vi "Move Main VI Controls.vi"(8 "error in":errorcluster, 11 "VIRef in":refnum<vi>) -> (0 "error out":errorcluster)   [LabVIEW 2018]
uses:
  <vilib>/Utility/miscctls.llb/LVPointTypeDef.ctl
panel:
  out "Height":i16
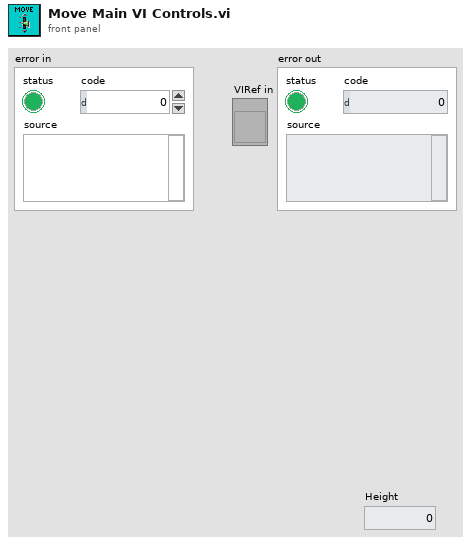
[diagram p1: front panel]
types:
  T1 = typedef "LVPointTypeDef.ctl" = cluster{"Horizontal":i16, "Vertical":i16}
  T2 = typedef "LVRectTypeDef.ctl" = cluster{"Left":i16, "Top":i16, "Right":i16, "Bottom":i16}
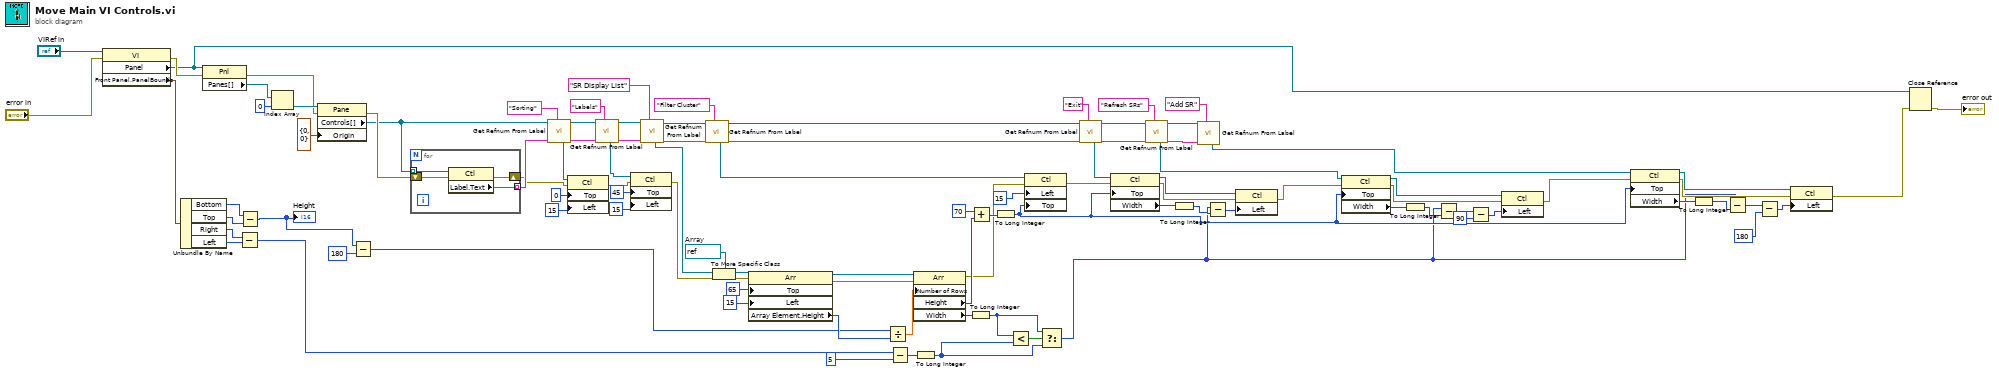
[diagram p0: block diagram]
diagram:
  w69 = refnum<vi> refnum  # Array
  n1 = property class="VI"(reference="VIRef in", error in="error in") -> (error out=w95:errorcluster, "Panel"=w9:refnum<vi>, "Front Panel.PanelBounds"=w92:T2)  [unwired: 1 out]
  n2 = Unbundle By Name(w92) -> ("Bottom"=w57:i16, "Top"=w56:i16, "Right"=w47:i16, "Left"=w46:i16)
  n3 = property class="Pnl"(reference=w9, error in=w95) -> (error out=w94:errorcluster, "Panes[]"=w96:refnum<vi>[])  [unwired: 1 out]
  n4 = Subtract(x=w47, y=w46) -> (x-y=w19:i16)
  n5 = Subtract(x=w57, y=w56) -> (x-y=w54:i16)
  "Height" <- w54
  n6 = Index Array(array=w96, index=0) -> (element=w97:refnum<vi>)
  n7 = property class="Pane"(reference=w97, error in=w94, "Origin"=T1 {"Horizontal"=0, "Vertical"=0}) -> (error out=w93:errorcluster, "Controls[]"=w90:refnum<vi>[])  [unwired: 1 out]
  n8 = Subtract(x=w54, y=i16 180) -> (x-y=w53:i16)
  n9 = for {
    tunnel: w90 -> [w102] mode=indexing
    shift-right: [w103] -> w62
    shift-left: w93 -> [w104]
    tunnel: [w101] -> w89 mode=indexing
    n10 = property class="Ctl"(reference=w102, error in=w104) -> (error out=w103:errorcluster, "Label.Text"=w101:string)  [unwired: 1 out]
  }
  n11 = call "Get Refnum From Label.vi"("label"="Sorting" ("element"), "label array in"=w89, "controls[] in"=w90) -> ("label array out"=w86:string[], "controls[] out"=w87:refnum<vi>[], "refnum out"=w72:refnum<vi>)  [unwired: 6 in]
  n12 = property class="Ctl"(reference=w72, error in=w62, "Top"=0 ("Position:Left"), "Left"=15 ("Position:Top")) -> (error out=w65:errorcluster)  [unwired: 1 out]
  n13 = call "Get Refnum From Label.vi"("label"="Labels" ("element"), "label array in"=w86, "controls[] in"=w87) -> ("label array out"=w83:string[], "controls[] out"=w84:refnum<vi>[], "refnum out"=w71:refnum<vi>)  [unwired: 6 in]
  n14 = property class="Ctl"(reference=w71, error in=w65, "Top"=45 ("Position:Top"), "Left"=15 ("Position:Left")) -> (error out=w64:errorcluster)  [unwired: 1 out]
  n15 = call "Get Refnum From Label.vi"("label"="SR Display List" ("element"), "label array in"=w83, "controls[] in"=w84) -> ("label array out"=w85:string[], "controls[] out"=w82:refnum<vi>[], "refnum out"=w3:refnum<vi>)  [unwired: 6 in]
  n16 = call "Get Refnum From Label.vi"("label"="Filter Cluster" ("element"), "label array in"=w85, "controls[] in"=w82) -> ("label array out"=w5:string[], "controls[] out"=w4:refnum<vi>[], "refnum out"=w52:refnum<vi>)  [unwired: 6 in]
  n17 = To More Specific Class(target class=w69, reference=w3, error in=w64) -> (specific class reference=w2:refnum<vi>, error out=w63:errorcluster)
  n18 = property class="Arr"(reference=w2, error in=w63, "Top"=65 ("Position:Top"), "Left"=15 ("Position:Left")) -> (reference out=w60:refnum<vi>, error out=w6:errorcluster, "Array Element.Height"=w59:u32)
  n19 = Divide(x=w53, y=w59) -> (x/y=w58:dbl)
  n20 = Subtract(x=w19, y=i16 5) -> (x-y=w16:i16)
  n21 = property class="Arr"(reference=w60, error in=w6, "Number of Rows"=w58) -> (error out=w45:errorcluster, "Height"=w50:u32, "Width"=w17:u32)  [unwired: 1 out]
  n22 = To Long Integer(number=w16) -> (32bit integer=w13:i32)
  n23 = To Long Integer(number=w17) -> (32bit integer=w14:i32)
  n24 = Add(x=u32 70, y=w50) -> (x+y=w48:u32)
  n25 = To Long Integer(number=w48) -> (32bit integer=w23:i32)
  n26 = Less?(x=w14, y=w13) -> (x < y?=w15:bool)
  n27 = property class="Ctl"(reference=w52, error in=w45, "Left"=15 ("Position:Left"), "Top"=w23) -> (error out=w11:errorcluster)  [unwired: 1 out]
  n28 = Select(t=w14, s=w15, f=w13) -> (s? t:f=w12:i32)
  n29 = call "Get Refnum From Label.vi"("label"="Exit" ("element"), "label array in"=w5, "controls[] in"=w4) -> ("label array out"=w73:string[], "controls[] out"=w76:refnum<vi>[], "refnum out"=w1:refnum<vi>)  [unwired: 6 in]
  n30 = property class="Ctl"(reference=w1, error in=w11, "Top"=w23) -> (reference out=w41:refnum<vi>, error out=w40:errorcluster, "Width"=w42:u32)
  n31 = call "Get Refnum From Label.vi"("label"="Refresh SRs" ("element"), "label array in"=w73, "controls[] in"=w76) -> ("label array out"=w74:string[], "controls[] out"=w75:refnum<vi>[], "refnum out"=w36:refnum<vi>)  [unwired: 6 in]
  n32 = To Long Integer(number=w42) -> (32bit integer=w22:i32)
  n33 = call "Get Refnum From Label.vi"("label"="Add SR" ("element"), "label array in"=w74, "controls[] in"=w75) -> ("refnum out"=w26:refnum<vi>)  [unwired: 6 in, 2 out]
  n34 = Subtract(x=w12, y=w22) -> (x-y=w43:i32)
  n35 = property class="Ctl"(reference=w41, error in=w40, "Left"=w43) -> (error out=w25:errorcluster)  [unwired: 1 out]
  n36 = property class="Ctl"(reference=w36, error in=w25, "Top"=w23) -> (reference out=w38:refnum<vi>, error out=w39:errorcluster, "Width"=w37:u32)
  n37 = To Long Integer(number=w37) -> (32bit integer=w21:i32)
  n38 = Subtract(x=w12, y=w21) -> (x-y=w35:i32)
  n39 = Subtract(x=w35, y=90) -> (x-y=w33:i32)
  n40 = property class="Ctl"(reference=w38, error in=w39, "Left"=w33) -> (error out=w24:errorcluster)  [unwired: 1 out]
  n41 = property class="Ctl"(reference=w26, error in=w24, "Top"=w23) -> (reference out=w28:refnum<vi>, error out=w27:errorcluster, "Width"=w29:u32)
  n42 = To Long Integer(number=w29) -> (32bit integer=w20:i32)
  n43 = Subtract(x=w12, y=w20) -> (x-y=w30:i32)
  n44 = Subtract(x=w30, y=180) -> (x-y=w32:i32)
  n45 = property class="Ctl"(reference=w28, error in=w27, "Left"=w32) -> (error out=w10:errorcluster)  [unwired: 1 out]
  n46 = Close Reference(reference=w9, error in (no error)=w10) -> (error out=→"error out":errorcluster)
